vi "Current_Time.vi"(11 "Current Time prev":dbl) -> (3 "Current Time":dbl)   [LabVIEW 2018]
doc: "This VI calculates current time by adding 0.1s to previous time value.\n\nInputs:\nCurrent time prev.\n\nOutputs:\nCurrent time."
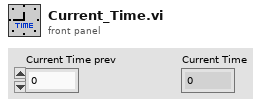
[diagram p1: front panel]
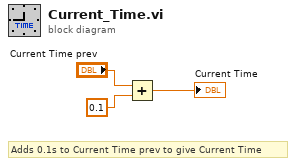
[diagram p0: block diagram]
diagram:
  # "Adds 0.1s to Current Time prev to give Current Time"
  n1 = Add(x="Current Time prev", y=0.1 ("x")) -> (x+y=→"Current Time":dbl)
